vi "Sort Path Groups By Rank.vi"(0 "Path Groups in":refnum<class "Path Group.lvclass">[](array[class]), 11 "error in (no error)":errorcluster) -> (4 "Path Groups out":refnum<class "Path Group.lvclass">[](array[class]), 15 "error out":errorcluster)   [LabVIEW 2023, in "RFCalAndFixtureCharact.Common.lvlib"]
uses:
  RFCalAndFixtureCharact.Common.lvlib
  Base Classes/Path Group/Path Group.lvclass
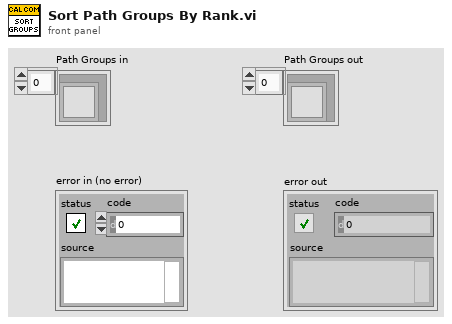
[diagram p1: front panel]
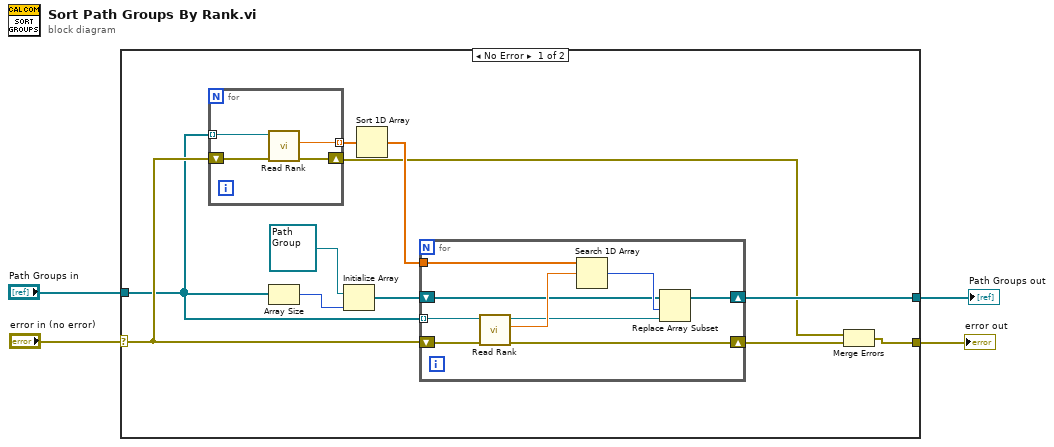
[diagram p0: block diagram]
diagram:
  n1 = case shown="No Error" "error in (no error)" {
    selector: "error in (no error)" -> [w9 w29]
    tunnel: "Path Groups in" -> [w5 w30]
    tunnel: [w10 w30] -> w2
    tunnel: [w7 w29] -> w1
    frame No Error {
      n2 = for {
        tunnel: w5 -> [w28] mode=indexing
        tunnel: [w27] -> w15 mode=indexing
        shift-right: [w25] -> w6
        shift-left: w9 -> [w26]
        n3 = call-dynamic "Read Rank.vi"("error in (no error)"=w26, "Path Group in"=w28) -> ("error out"=w25:errorcluster, "Rank"=w27:dbl)  [unwired: 7 in, 1 out]
      }
      n4 = Array Size(array=w5) -> (size(s)=w14:i32)
      n5 = Initialize Array(refnum<class "Path Group.lvclass"> refnum ("Calibration Common.lvlib:Path Group.lvclass"), w14) -> (w11:refnum<class "Path Group.lvclass">[])
      n6 = Sort 1D Array(array=w15) -> (sorted array=w12:dbl[])
      n7 = for {
        tunnel: w5 -> [w24] mode=indexing
        tunnel: w12 -> [w23]
        shift-right: [w18] -> w10
        shift-left: w11 -> [w20]
        shift-right: [w16] -> w8
        shift-left: w9 -> [w17]
        n8 = call-dynamic "Read Rank.vi"("error in (no error)"=w17, "Path Group in"=w24) -> ("error out"=w16:errorcluster, "Rank"=w22:dbl, "Path Group out"=w19:refnum<class "Path Group.lvclass">)  [unwired: 7 in]
        n9 = Search 1D Array(1D array=w23, element=w22) -> (index of element=w21:i32)  [unwired: 1 in]
        n10 = Replace Array Subset(array=w20, new element=w19, index=w21) -> (w18:refnum<class "Path Group.lvclass">[])
      }
      n11 = Merge Errors(w6, w8) -> (w7:errorcluster)
    }
    frame Error {
    }
  }
  "error out" <- w1
  "Path Groups out" <- w2
